vi "sub_ofdm_cp_removed.vi"(9 "CP length":i32=64, 11 "time ofdm symbol":cdb[](array[numeric])) -> (3 "cp removed ofdm symbol":cdb[](array[numeric]))   [LabVIEW 2014]
panel:
  out "output size":i32
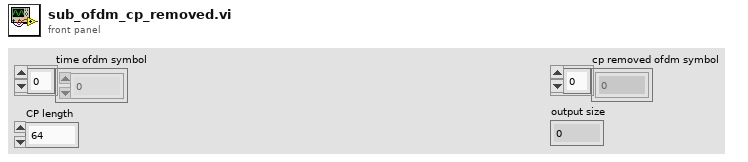
[diagram p1: front panel]
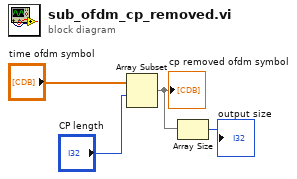
[diagram p0: block diagram]
diagram:
  n1 = Array Subset(array="time ofdm symbol", index="CP length") -> (w2:cdb[])  [unwired: 1 in]
  "cp removed ofdm symbol" <- w2
  n2 = Array Size(array=w2) -> (size(s)=→"output size":i32)
